vi "get_continuous_samples.vi"(8 "error in (no error)":errorcluster, 11 "GenericWriteSignals.lvclass in":refnum<class "GenericSignalWriter.lvclass">) -> (0 "error out":errorcluster, 2 "continuous samples":i32, 3 "GenericWriteSignals.lvclass out":refnum<class "GenericSignalWriter.lvclass">)   [LabVIEW 2010, in "GenericSignalWriter.lvclass"]
uses:
  GenericSignalWriter.lvclass
  GenericSignalWriter.lvclass/GenericSignalWriter.ctl
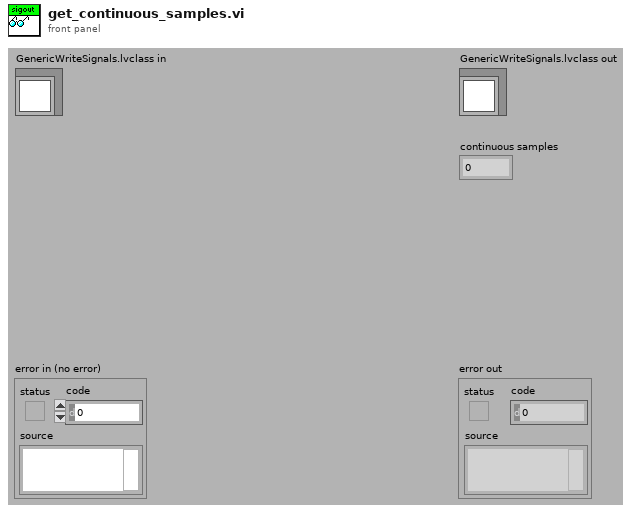
[diagram p1: front panel]
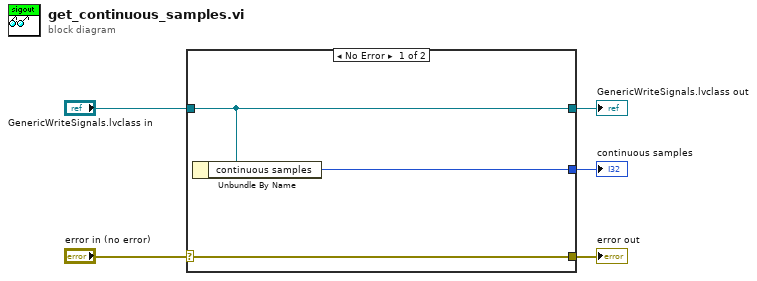
[diagram p0: block diagram]
diagram:
  n1 = case shown="No Error" "error in (no error)" {
    selector: "error in (no error)" -> [w8 w9]
    tunnel: [w8 w9] -> w4
    tunnel: [w7 w10] -> w2
    tunnel: "GenericWriteSignals.lvclass in" -> [w7 w10]
    tunnel: [w6 _] -> w1
    frame No Error {
      n2 = Unbundle By Name(w7) -> ("continuous samples"=w6:i32)
    }
    frame Error {
    }
  }
  "error out" <- w4
  "GenericWriteSignals.lvclass out" <- w2
  "continuous samples" <- w1
